vi "Set Actuator Position.vi"(0 "Setpoint from Home":dbl) -> ()   [LabVIEW 2012]
uses:
  Globals/Actuator Home Position.vi
  Globals/Jaguar Commands.vi
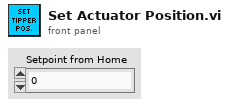
[diagram p1: front panel]
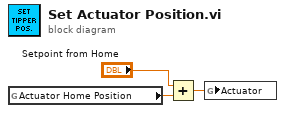
[diagram p0: block diagram]
diagram:
  n1 = global read "Actuator Home Position.vi" "Actuator Home Position"() -> (w3:dbl)
  n2 = Add(x="Setpoint from Home", y=w3) -> (x+y=w2:dbl)
  n3 = global write "Jaguar Commands.vi" "Actuator"(w2) -> ()
